vi "Excel Example.vi"() -> ()   [LabVIEW 2019]
panel:
  out "data":string[][](array[string])
  out "array":dbl[][][](array[numeric])
  in  "Array":path[](array[path])
  in  "Start and End":T1
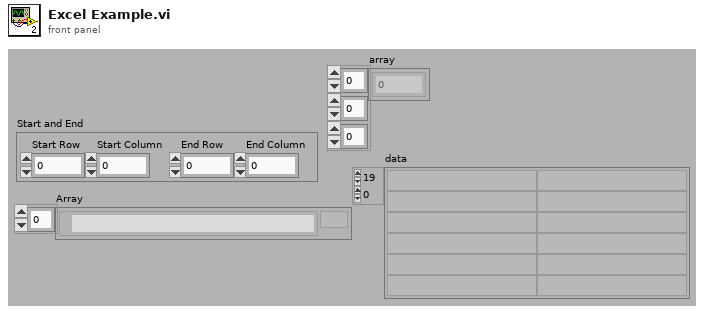
[diagram p1: front panel]
types:
  T1 = cluster{"Start Row":i32, "Start Column":i32, "End Row":i32, "End Column":i32}
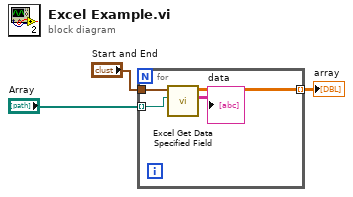
[diagram p0: block diagram]
diagram:
  n1 = for {
    tunnel: "Start and End" -> [w7]
    tunnel: "Array" -> [w6] mode=indexing
    tunnel: [w5] -> w1 mode=indexing
    n2 = call "Excel Get Data Specified Field.vi"("path"=w6, "Start and End"=w7) -> ("data"=→"data":string[][], "array"=w5:dbl[][])  [unwired: 3 in, 1 out]
  }
  "array" <- w1
